vi "OAT Orbit Plot (Vector Data).vi"(0 "magnitudes":T4(array[cluster]) {"magnitude" format="%.2f"; "time/rev/rpm" format="%.2f"}, 1 "orbit plot ref":refnum<vi>, 2 "order to display":dbl=1.0 format="%.2f", 3 "max axis display value":dbl format="%.2f", 5 "phases [phase lag]":cluster{"time/rev/rpm":dbl[], "phase":dbl[]}[](array[cluster]) {"phase" format="%.2f"; "time/rev/rpm" format="%.2f"}, 7 "samples/rev wanted":i32=64, 9 "revolutions to display [rev]":cluster{"start":dbl, "duration":dbl}={"start"=0.0, "duration"=1.0} {"duration" format="%.2f"; "start" format="%.2f"}, 11 "error in (no error)":errorcluster, 12 "channel settings":T1={"shaft rotating direction"=0, "probe angles [deg]"={"X"=0, "Y"=90}} {"probe angles [deg]"."Y" max=360 step=1; "probe angles [deg]"."X" max=360 step=1; "shaft rotating direction" items=["CCW", "CW"]}, 13 "view":T3={"dB on? (F)"=FALSE, "unwrap phase? (T)"=TRUE, "unit in degree? (T)"=TRUE}, 14 "trigger pulse direction":u16(ring)=1 items=["positive going", "negative going"]) -> (4 "orbit plot":T2, 10 "orbit precession direction":u16(ring) items=["forward", "backward"], 15 "error out":errorcluster)   [LabVIEW 2017]
doc: "Draws an orbit plot on an XY graph. You can use this polymorphic VI to draw an orbit plot with unfiltered or filtered data. Unfiltered data comes from the <B>even angle signals</B> input, filtered data from the <B>magnitudes</B> and <B>phases [phase lag]</B> inputs. The data type you wire to the <B>even angle signals</B> input determines the polymorphic instance to use."
uses:
  <vilib>/addons/Sound and Vibration/Order Analysis/Backward Compatibility/SubVIs/oa_Orbit Plot Control.ctl
  <vilib>/addons/Sound and Vibration/Order Analysis/Resample Order Tracking/SoundVib_Resampling.lvlib
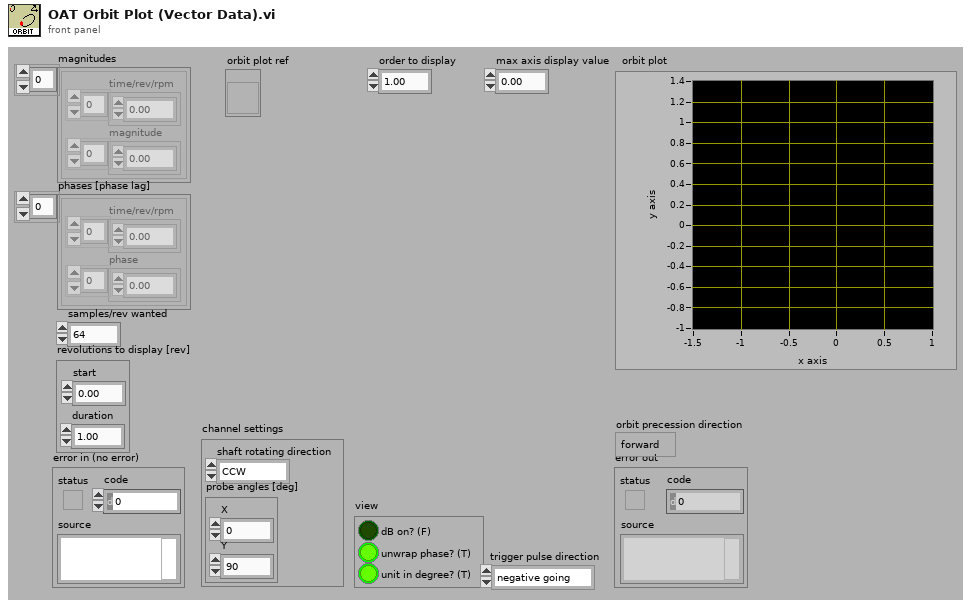
[diagram p1: front panel]
types:
  T1 = cluster{"shaft rotating direction":u16, "probe angles [deg]":cluster{"X":u32, "Y":u32}}
  T2 = typedef "oa_Orbit Plot Control.ctl" = cluster{dbl[], dbl[]}[]
  T3 = cluster{"dB on? (F)":bool, "unwrap phase? (T)":bool, "unit in degree? (T)":bool}
  T4 = cluster{"time/rev/rpm":dbl[], "magnitude":dbl[]}[]
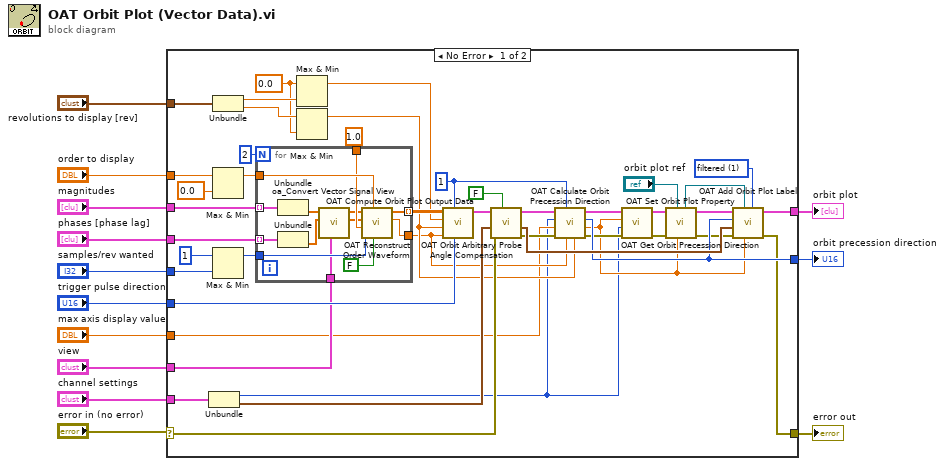
[diagram p0: block diagram]
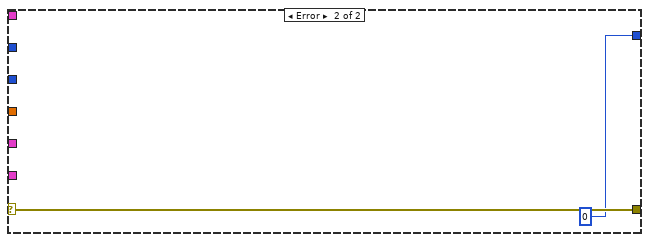
[diagram p2: hidden frame]
diagram:
  n1 = case shown="No Error" "error in (no error)" {
    selector: "error in (no error)" -> [w28 w72]
    tunnel: "order to display" -> [w19 _]
    tunnel: "magnitudes" -> [w56 _]
    tunnel: "phases [phase lag]" -> [w55 _]
    tunnel: "view" -> [w20 _]
    tunnel: "revolutions to display [rev]" -> [w53 _]
    tunnel: [w50 _] -> w5
    tunnel: [w25 w72] -> w8
    tunnel: [w29 u16 0 ("orbit precession direction")] -> w7
    tunnel: "samples/rev wanted" -> [w44 _]
    tunnel: "trigger pulse direction" -> [w33 _]
    tunnel: "max axis display value" -> [w16 _]
    tunnel: "channel settings" -> [w31 _]
    frame No Error {
      w34 = u16 1 items=["unfiltered", "filtered"] ("plot type")
      w47 = 0.0 ("t")
      w35 = 1 ("tach duty")
      n2 = Unbundle(w31) -> ("shaft rotating direction"=w14:u16, "probe angles [deg]"=w30:cluster{"X":u32, "Y":u32})
      n3 = Unbundle(w53) -> ("start"=w52:dbl, "duration"=w48:dbl)
      n4 = Max & Min(x=w19, y=0.0 ("t")) -> (max(x,y)=w18:dbl)  [unwired: 1 out]
      n5 = Max & Min(x=1, y=w44) -> (max(x,y)=w42:i32)  [unwired: 1 out]
      n6 = for {
        N: 2 -> [_]
        tunnel: [w70] -> w54 mode=indexing
        tunnel: w18 -> [w69]
        tunnel: 1.0 ("y") -> [w68]
        tunnel: w56 -> [w67] mode=indexing
        tunnel: w55 -> [w66] mode=indexing
        tunnel: [w65] -> w23
        tunnel: w42 -> [w64]
        tunnel: w20 -> [w59]
        n7 = Unbundle(w67) -> ("magnitude"=w62:dbl[])  [unwired: 1 out]
        n8 = Unbundle(w66) -> ("phase"=w61:dbl[])  [unwired: 1 out]
        n9 = call <vilib>:"oa_Convert Vector Signal View.vi"("view"=w59, "phase"=w61, "magnitude"=w62) -> ("phase out"=w60:dbl[], "magnitude out"=w63:dbl[])  [unwired: 7 in]
        n10 = call <vilib>:"OAT Reconstruct Order Waveform.vi"("unit in degree? (F)"=FALSE, "order"=w69, "samples/revolution wanted"=w64, "samples/revolution"=w68, "phase lag"=w60, "magnitude"=w63) -> ("actual samples/rev"=w65:dbl, "order waveform"=w70:dbl[])  [unwired: 3 in, 1 out]
      }
      n11 = Max & Min(x=w47, y=w52) -> (max(x,y)=w49:dbl)  [unwired: 1 out]
      n12 = Max & Min(x=w48, y=w47) -> (max(x,y)=w24:dbl)  [unwired: 1 out]
      n13 = call <vilib>:"OAT Compute Orbit Plot Output Data.vi"("trigger pulse direction"=w33, "tach duty"=w35, "actual samples/rev"=w23, "revolutions"=w24, "start"=w49, "order waveform"=w54) -> ("orbit data"=w51:cluster{dbl[], dbl[]}[])  [unwired: 5 in]
      n14 = call <vilib>:"OAT Orbit Arbitrary Probe Angle Compensation.vi"("select methods"=FALSE, "error in (no error)"=w28, "probe angle"=w30, "XY plot data in"=w51) -> ("error out"=w22:errorcluster, "probe angle out"=w46:cluster{"X (red)":dbl, "Y (blue)":dbl}, "XY plot data out"=w41:cluster{dbl[], dbl[]}[])  [unwired: 5 in]
      n15 = call <vilib>:"OAT Calculate Orbit Precession Direction.vi"("revolutions"=w24, "actual samples/rev"=w23, "tach duty"=w35, "error in (no error)"=w22, "max axis value"=w16, "shaft rotating direction"=w14, "XY plot data in"=w41) -> ("error out"=w21:errorcluster, "max value"=w15:dbl, "orbit precession direction"=w29:u16, "XY plot data out"=w40:cluster{dbl[], dbl[]}[])  [unwired: 1 in]
      n16 = call <vilib>:"OAT Get Orbit Precession Direction.vi"("error in (no error)"=w21, "shaft rotating direction"=w14, "max data value"=w15, "XY plot data in"=w40) -> ("error out"=w27:errorcluster, "XY plot data out"=w39:cluster{dbl[], dbl[]}[])  [unwired: 6 in]
      n17 = call <vilib>:"OAT Set Orbit Plot Property.vi"("max value"=w15, "orbit plot ref"="orbit plot ref", "error in (no error)"=w27, "XY plot data in"=w39) -> ("error out"=w26:errorcluster, "XY plot data out"=w38:cluster{dbl[], dbl[]}[], "orbit plot ref"=w36:refnum<vi>)  [unwired: 5 in]
      n18 = call <vilib>:"OAT Add Orbit Plot Label.vi"("plot type"=w34, "max value"=w15, "orbit plot ref"=w36, "error in (no error)"=w26, "probe angle out"=w46, "orbit precession direction"=w29, "XY plot data in"=w38) -> ("error out"=w25:errorcluster, "XY plot data out"=w50:cluster{dbl[], dbl[]}[])  [unwired: 3 in]
    }
    frame Error {
    }
  }
  "error out" <- w8
  "orbit precession direction" <- w7
  "orbit plot" <- w5
